vi "RGB to Color.vi"(1 "B":u16, 2 "G":u16, 3 "R":u16) -> (0 "Color":u32(colorbox))   [LabVIEW 2015]
doc: "Converts a red, green, and blue value from 0 to 255 to the corresponding RGB color."
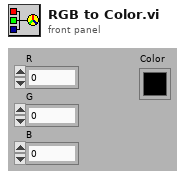
[diagram p1: front panel]
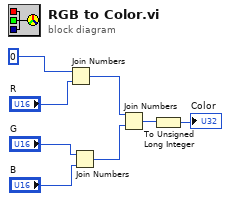
[diagram p0: block diagram]
diagram:
  n1 = Join Numbers(hi=u16 0, lo="R") -> ((hi.lo)=w4:u32)
  n2 = Join Numbers(hi="G", lo="B") -> ((hi.lo)=w3:u32)
  n3 = Join Numbers(hi=w4, lo=w3) -> ((hi.lo)=w2:u64)
  n4 = To Unsigned Long Integer(number=w2) -> (unsigned 32bit integer=→"Color":u32)
